vi "WidthRectagle.vi"(11 "xInput":i16) -> (3 "xOutput":i16)   [LabVIEW 2014]
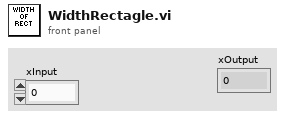
[diagram p1: front panel]
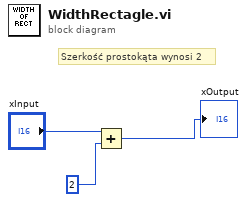
[diagram p0: block diagram]
diagram:
  # "Szerkość prostokąta wynosi 2"
  n1 = Add(x="xInput", y=i16 2) -> (x+y=→"xOutput":i16)
